vi "Cross_Correlation_normalised.vi"() -> ()   [LabVIEW 2018]
uses:
  <vilib>/Instr/_visa.llb/VISA Open Access Mode.ctl
  <vilib>/express/express signal manip/GetorSetDDTAttributes/Shared VIs/TimeType.ctl
  <vilib>/Analysis/2dsp.llb/1D Auto Correlation (DBL).vi
  <vilib>/Instr/_visa.llb/VISA Configure Serial Port (Instr).vi
  <vilib>/Analysis/2dsp.llb/1D Cross Correlation (DBL).vi
  <vilib>/express/express signal manip/GetorSetDDTAttributes/Shared VIs/TimeMode Enum to Boolean.vi
  <vilib>/express/express shared/transition.llb/Dynamic To Waveform Array.vi
  <vilib>/express/express signal manip/GetorSetDDTAttributes/Set DDT Attributes/SetT0.vi
  <vilib>/express/express shared/transition.llb/Waveform Array To Dynamic.vi
  <vilib>/express/express signal manip/GetorSetDDTAttributes/Set DDT Attributes/Set DDT Properties.xnode
  <vilib>/express/express signal manip/GetorSetDDTAttributes/Shared VIs/GetSetShared.lvlib
  <vilib>/Analysis/NI_AALPro.lvlib
panel:
  out "x*y":dbl
  out "max index(es)":i32
  out "max":dbl
  out "max value":dbl
  out "size":i32
  out "Waveform Graph":dbl[](graph)
  out "max index":i32
  out "x-y 3":u32
  out "Delay (ms)":i32
  out "GF min":dbl
  out "GF max":dbl
  out "LF min":dbl
  out "LF max":dbl
  out "x .or. y?":bool
  out "Grip Force":dynamicdata(graph)
  out "Load Force":dynamicdata(graph)
  in  "?":bool
  in  "Access Mode":T1 items=["VISA Defaults"=0, "Exclusive Lock"=1, "Load Configured Settings"=4]
  in  "data bits (8)":u16=8 min=5 max=8 step=1
  out "error out":errorcluster
  in  "byte count":u32=1000
  in  "error in (no error)":errorcluster
  in  "VISA resource name":refnum<visa-resource-name>="COM3"
  in  "baud rate (9600)":u32=38400
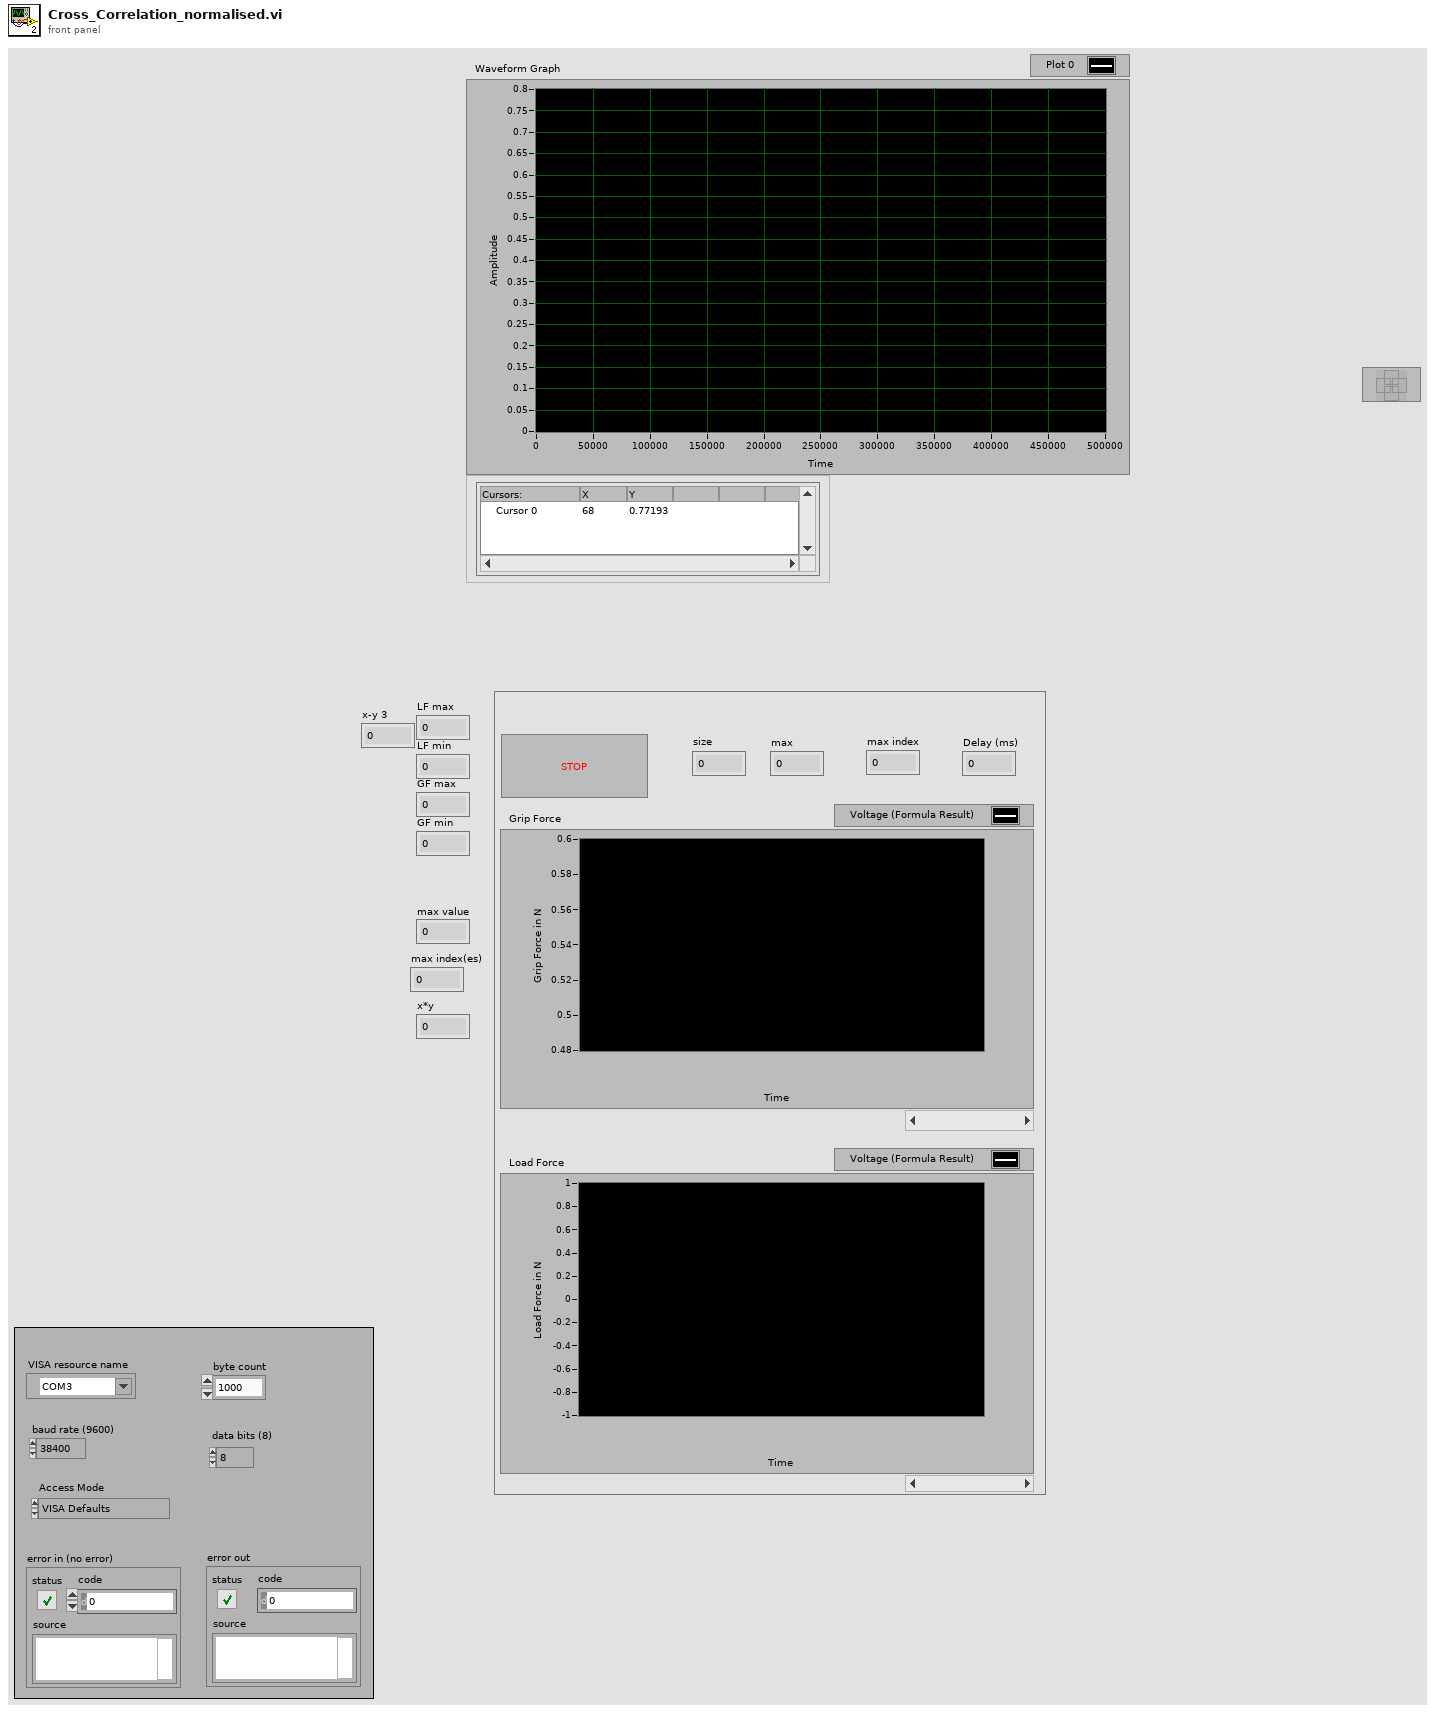
[diagram p1: front panel]
types:
  T1 = typedef "VISA Open Access Mode.ctl" = u32
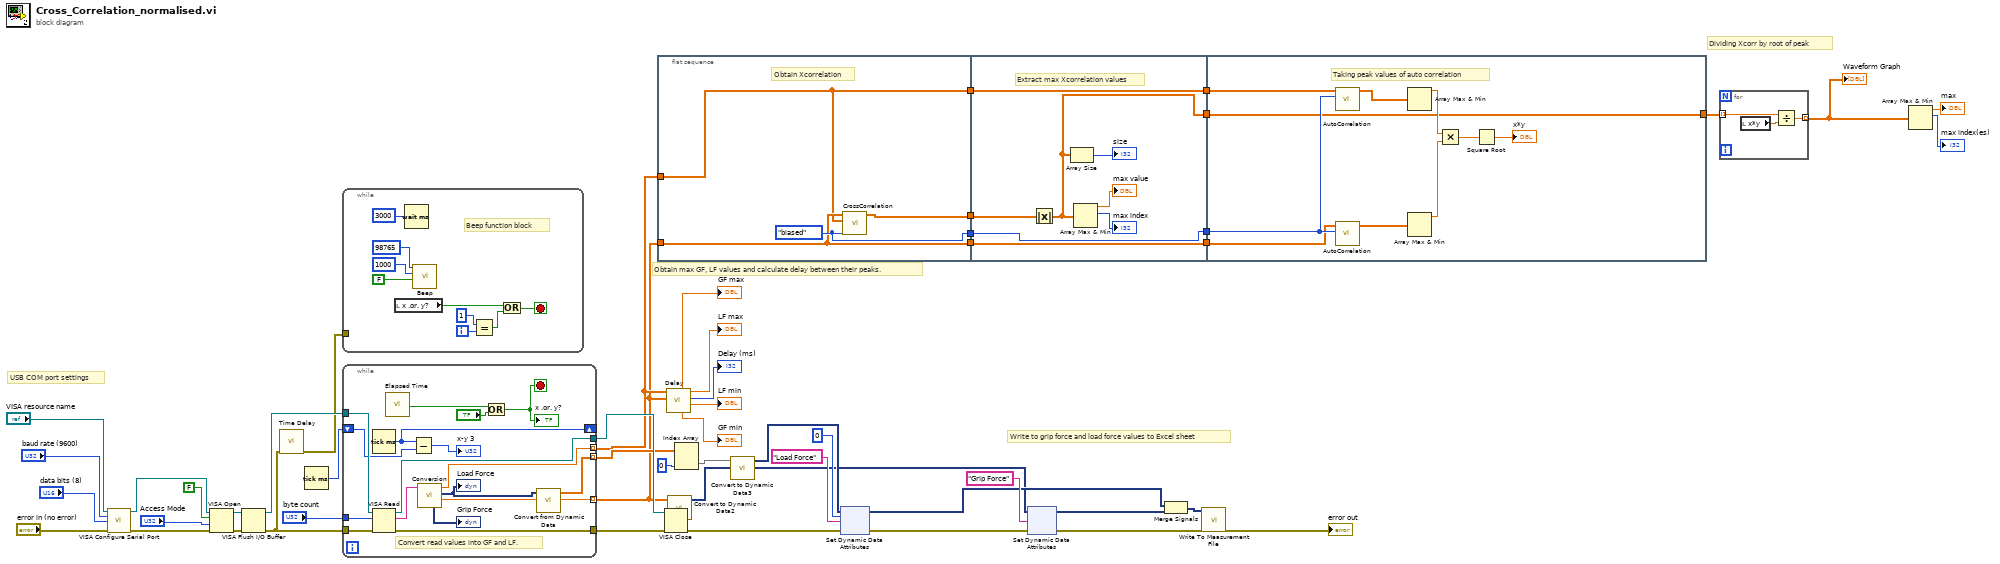
[diagram p0: block diagram]
diagram:
  # "Obtain max GF, LF values and calculate delay between their peaks."
  # "Write to grip force and load force values to Excel sheet"
  # "USB COM port settings"
  # "Dividing Xcorr by root of peak"
  n1 = call-poly "VISA Configure Serial Port"("VISA resource name"="VISA resource name", "baud rate (9600)"="baud rate (9600)", "data bits (8)"="data bits (8)", "error in (no error)"="error in (no error)") -> ("VISA resource name out"=w47:refnum<visa-resource-name>, "error out"=w50:errorcluster)  [unwired: 10 in]
  n2 = VISA Open(duplicate session (F)=FALSE, access mode="Access Mode", error in (no error)=w50, VISA resource name=w47) -> (VISA resource name=w41:refnum<visa-resource-name>, error out=w40:errorcluster)  [unwired: 1 in]
  n3 = VISA Flush I/O Buffer(VISA resource name=w41, error in (no error)=w40) -> (VISA resource name out=w39:refnum<visa-resource-name>, error out=w37:errorcluster)  [unwired: 1 in]
  n4 = call "Time Delay"("error in (no error)"=w37) -> ("error out"=w36:errorcluster)  [unwired: 10 in]
  n5 = Tick Count (ms)() -> (millisecond timer value=w23:u32)
  n6 = while {
    tunnel: w36 -> [_]
    i -> [w56]
    stop <- w52 stop-if-true
    # "Beep function block"
    n7 = local read "x .or. y?"() -> (w54:bool)
    n8 = Wait (ms)(milliseconds to wait=u32 3000) -> ()  [unwired: 1 out]
    n9 = call <vilib>:"Beep.vi"("use system alert? (T)"=FALSE, "duration (msec)"=u32 1000, "frequency (Hz)"=u32 98765) -> ()  [unwired: 9 in]
    n10 = Equal?(x=1, y=w56) -> (x = y?=w53:bool)
    n11 = Or(x=w54, y=w53) -> (x .or. y?=w52:bool)
  }
  n12 = while {
    tunnel: "byte count" -> [w76]
    tunnel: w39 -> [w75]
    tunnel: w37 -> [w77]
    tunnel: [w74] -> w42
    tunnel: [w69] -> w38
    tunnel: [w66] -> w25 mode=indexing
    shift-right: [w65] -> _
    shift-left: w23 -> [w64]
    tunnel: [w62] -> w12 mode=indexing
    tunnel: [w61] -> w13 mode=indexing
    stop <- w71 stop-if-true
    # "Convert read values into GF and LF."
    n13 = Tick Count (ms)() -> (millisecond timer value=w65:u32)
    n14 = VISA Read(VISA resource name=w75, byte count=w76, error in (no error)=w77) -> (VISA resource name out=w69:refnum<visa-resource-name>, read buffer=w70:string, error out=w74:errorcluster)  [unwired: 1 out]
    n15 = call "Elapsed Time"() -> ("Time has Elapsed"=w73:bool)  [unwired: 12 in, 7 out]
    n16 = Subtract(x=w65, y=w64) -> (x-y=→"x-y 3":u32)
    n17 = call "Conversion.vi"("read buffer"=w70) -> ("GF"=w62:dbl, "Load Force"=w67:dynamicdata, "LF"=w61:dbl, "Grip Force"=→"Grip Force":dynamicdata)  [unwired: 7 in]
    "Load Force" <- w67
    n18 = Or(x=w73, y="?") -> (x .or. y?=w71:bool)
    "x .or. y?" <- w71
    n19 = call "Convert from Dynamic Data"("Dynamic Data Type"=w67) -> ("Array"=w66:dbl[])  [unwired: 3 in]
  }
  n20 = flat-sequence {
    tunnel: [w81] -> w14
    tunnel: w13 -> [w78]
    tunnel: w12 -> [w79]
    tunnel: [w79] -> w11
    tunnel: [w78] -> w10
    tunnel: [w80] -> w9
    tunnel: w14 -> [w88]
    tunnel: w11 -> [w83]
    tunnel: w10 -> [w86]
    tunnel: w9 -> [w87]
    tunnel: [w87] -> w8
    tunnel: [w86] -> w7
    tunnel: [w83] -> w6
    tunnel: [w82] -> w2
    tunnel: w8 -> [w98]
    tunnel: w7 -> [w99]
    tunnel: w6 -> [w97]
    tunnel: [w90] -> w3
    tunnel: w2 -> [w90]
    frame #0 {
      w80 = enum32{"none", "unbiased", "biased"}."biased" ("normalization")
      # "Obtain Xcorrelation"
      n21 = call-poly <vilib>:"CrossCorrelation.vi"("normalization"=w80, "Y"=w78, "X"=w79) -> ("Rxy"=w81:dbl[])  [unwired: 7 in, 1 out]
    }
    frame #1 {
      # "Extract max Xcorrelation values"
      n22 = Absolute Value(x=w88) -> (abs(x)=w82:dbl[])
      n23 = Array Size(array=w82) -> (size(s)=→"size":i32)
      n24 = Array Max & Min(array=w82) -> (max value=→"max value":dbl, max index (indices)=→"max index":i32)  [unwired: 2 out]
    }
    frame #2 {
      # "Taking peak values of auto correlation"
      n25 = call-poly <vilib>:"AutoCorrelation.vi"("normalization"=w98, "X"=w99) -> ("Rxx"=w96:dbl[])  [unwired: 8 in, 1 out]
      n26 = call-poly <vilib>:"AutoCorrelation.vi"("normalization"=w98, "X"=w97) -> ("Rxx"=w95:dbl[])  [unwired: 8 in, 1 out]
      n27 = Array Max & Min(array=w96) -> (max value=w94:dbl)  [unwired: 3 out]
      n28 = Array Max & Min(array=w95) -> (max value=w93:dbl)  [unwired: 3 out]
      n29 = Multiply(x=w94, y=w93) -> (x*y=w92:dbl)
      n30 = Square Root(x=w92) -> (sqrt(x)=→"x*y":dbl)
    }
  }
  n31 = VISA Close(VISA resource name=w38, error in (no error)=w42) -> (error out=w32:errorcluster)
  n32 = call "Delay.vi"("GF array"=w12, "LF array"=w13) -> ("LF min"=→"LF min":dbl, "Delay"=→"Delay (ms)":i32, "LF max"=→"LF max":dbl, "GF min"=→"GF min":dbl, "GF max"=→"GF max":dbl)  [unwired: 5 in]
  n33 = call "Convert to Dynamic Data2"("Array"=w12) -> ("Dynamic Data Type"=w16:dynamicdata)  [unwired: 3 in]
  n34 = Index Array(array=w25, index (col)=0 ("disabled index (col)")) -> (element=w17:dbl[])  [unwired: 1 in]
  n35 = call "Convert to Dynamic Data3"("Array"=w17) -> ("Dynamic Data Type"=w26:dynamicdata)  [unwired: 3 in]
  n36 = xnode "Set Dynamic Data Attributes"("Signals In"=w26, "error in"=w32, "Signal Index"=0, "Signal Name"="Load Force") -> ("Signals Out"=w30:dynamicdata, "error out"=w31:errorcluster)  [unwired: 1 in]
  n37 = xnode "Set Dynamic Data Attributes"("Signals In"=w16, "error in"=w31, "Signal Name"="Grip Force") -> ("Signals Out"=w29:dynamicdata, "error out"=w27:errorcluster)  [unwired: 2 in]
  n38 = Merge Signals(w30, w29) -> (w28:dynamicdata)
  n39 = call "Write To Measurement File"("Signals"=w28, "error in (no error)"=w27) -> ("error out"=→"error out":errorcluster)  [unwired: 15 in, 2 out]
  n40 = for {
    tunnel: w3 -> [w102] mode=indexing
    tunnel: [w101] -> w1 mode=indexing
    n41 = local read "x*y"() -> (w100:dbl)
    n42 = Divide(x=w102, y=w100) -> (x/y=w101:dbl)
  }
  "Waveform Graph" <- w1
  n43 = Array Max & Min(array=w1) -> (max value=→"max":dbl, max index (indices)=→"max index(es)":i32)  [unwired: 2 out]
